vi "test - breakdown and compact.vi"(8 "error in (no error)":errorcluster, 11 "TestCase in":refnum<class "testcase-Basic-Function.lvclass">) -> (0 "error out":errorcluster, 3 "TestCase out":refnum<class "testcase-Basic-Function.lvclass">)   [LabVIEW 2017, in "testcase-Basic-Function.lvclass"]
uses:
  testcase-Basic-Function.lvclass
  <vilib>/addons/_JKI Toolkits/VI Tester/TestCase.llb/TestCase.lvclass
  user.lib/_NEVSTOP/Communicable State Machine(CSM)/Communicable State Machine.lvlib
  C:/Program Files (x86)/National Instruments/LabVIEW 2017/vi.lib/addons/_JKI Toolkits/VI Tester/TestCase.llb/TestCase.lvclass
panel:
  out "States 2":string
  out "States":string
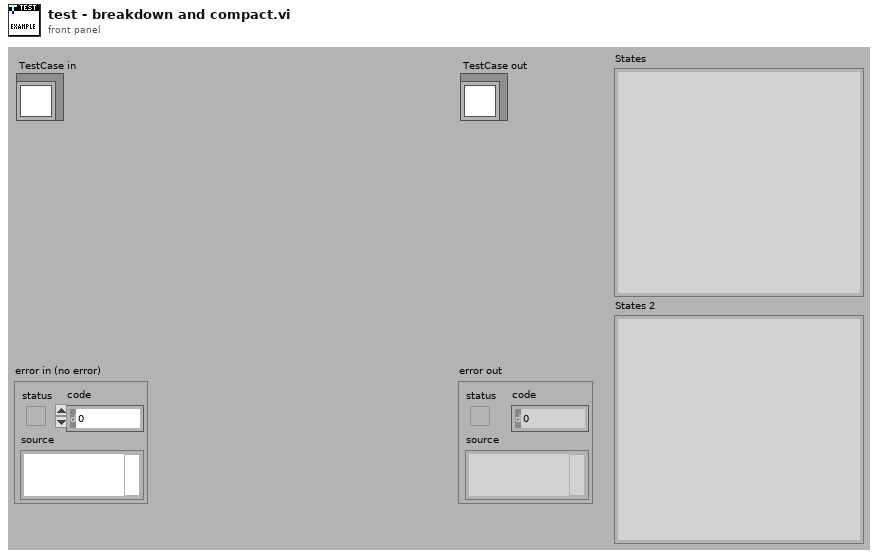
[diagram p1: front panel]
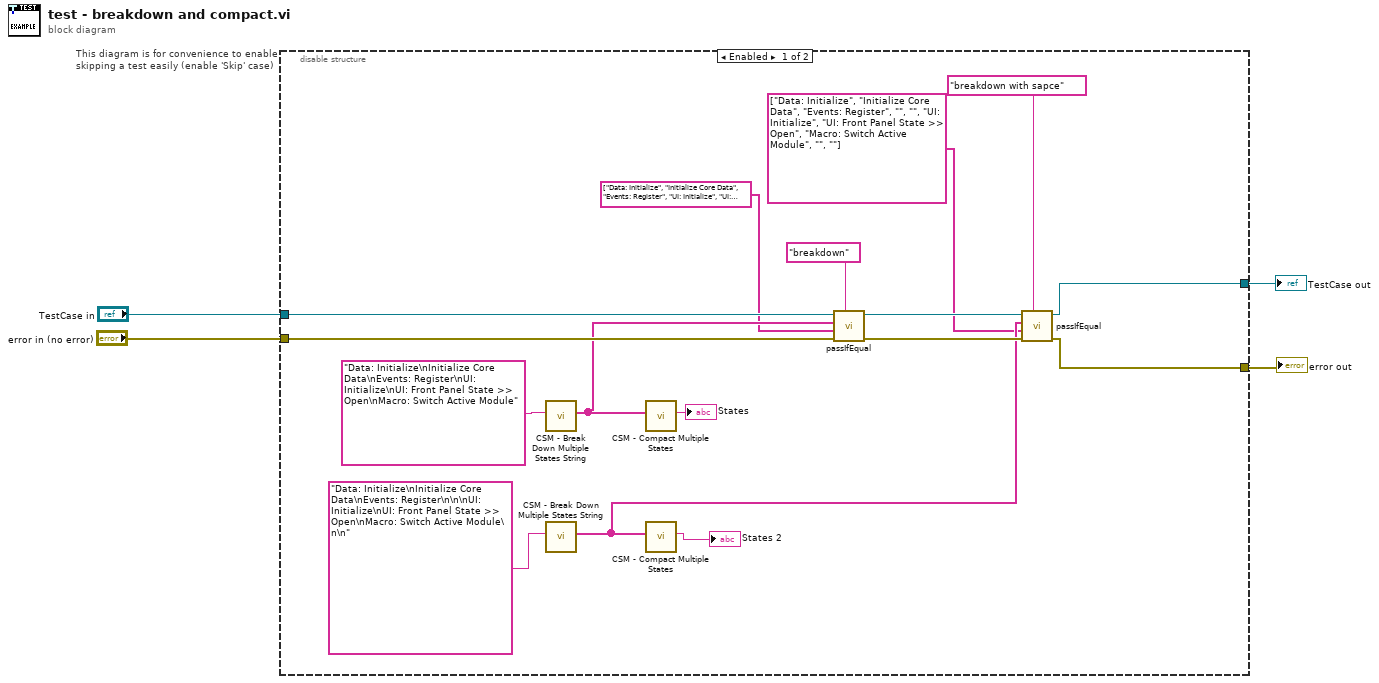
[diagram p0: block diagram]
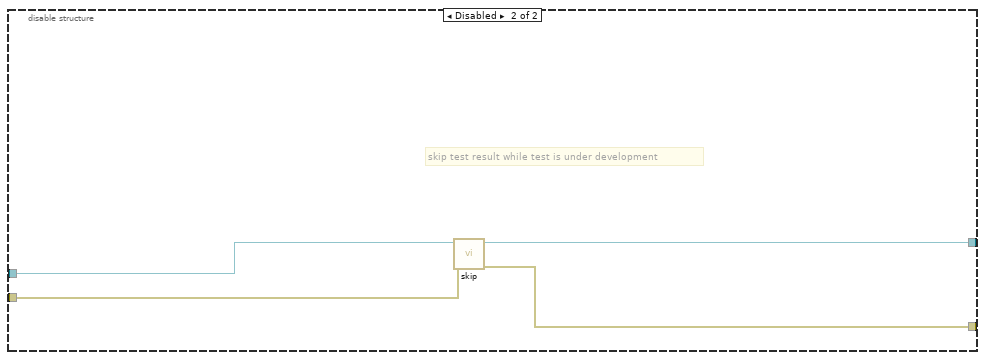
[diagram p2: hidden frame]
diagram:
  n1 = disable-structure "This diagram is for convenience to enable skipping a test easily (enable 'Skip' case)" shown="Enabled" {
    disable-tunnel: "TestCase in" -> [w20 w24]
    disable-tunnel: [w12 w22] -> w1
    disable-tunnel: [w11 w23] -> w3
    disable-tunnel: "error in (no error)" -> [w19 w21]
    frame Enabled {
      n2 = call "CSM - Break Down Multiple States String.vi"("States"="Data: Initialize\nInitialize Core Data\nEvents: Register\nUI: Initialize\nUI: Front Panel State >> Open\nMacro: Switch Active Module") -> ("Multiple States"=w18:string[])  [unwired: 10 in]
      n3 = call "CSM - Break Down Multiple States String.vi"("States"="Data: Initialize\nInitialize Core Data\nEvents: Register\n\n\nUI: Initialize\nUI: Front Panel State >> Open\nMacro: Switch Active Module\n\n" ("States 4")) -> ("Multiple States"=w10:string[])  [unwired: 10 in]
      n4 = call "CSM - Compact Multiple States.vi"("Multiple States"=w18) -> ("States"=→"States":string)  [unwired: 9 in]
      n5 = call "CSM - Compact Multiple States.vi"("Multiple States"=w10) -> ("States"=→"States 2":string)  [unwired: 9 in]
      n6 = call-dynamic "passIfEqual.vi"("custom report message (\"\")"="breakdown" ("custom report message (\"\")"), "error in (no error)"=w19, "y"=string[] ["Data: Initialize", "Initialize Core Data", "Events: Register", "UI: Initialize", "UI: Front Panel State >> Open", "Macro: Switch Active Module"] ("Multiple States"), "x"=w18, "TestCase in"=w20) -> ("error out"=w16:errorcluster, "TestCase out"=w15:refnum<class "testcase-Basic-Function.lvclass">)  [unwired: 5 in]
      n7 = call-dynamic "passIfEqual.vi"("custom report message (\"\")"="breakdown with sapce" ("custom report message (\"\")"), "error in (no error)"=w16, "y"=string[] ["Data: Initialize", "Initialize Core Data", "Events: Register", "", "", "UI: Initialize", "UI: Front Panel State >> Open", "Macro: Switch Active Module", "", ""] ("Multiple States 2"), "x"=w10, "TestCase in"=w15) -> ("error out"=w11:errorcluster, "TestCase out"=w12:refnum<class "testcase-Basic-Function.lvclass">)  [unwired: 5 in]
    }
    frame Disabled {
      # "skip test result while test is under development"
      n8 = call <vilib>:"skip.vi"("error in (no error)"=w21, "TestCase in"=w24) -> ("error out"=w23:errorcluster, "TestCase out"=w22:refnum<class "testcase-Basic-Function.lvclass">)  [unwired: 8 in]
    }
  }
  "error out" <- w3
  "TestCase out" <- w1
